vi "Config Parse.vi"(0 "Config File Path":path=path "C:/Automation/Configurations/VALEW.config", 11 "Error In":errorcluster) -> (4 "Pass/Fail?":bool, 6 "Report Text":string, 8 "VALEW_config":T1, 15 "Error Out":errorcluster)   [LabVIEW 2018, in "TL27.lvlib"]
uses:
  Projects/TL27.lvlib
  type defs/Config.ctl
  <vilib>/Utility/config.llb/Read Key (String).vi
  <vilib>/Utility/config.llb/Read Key (Boolean).vi
  <vilib>/Utility/config.llb/NI_LVConfig.lvlib
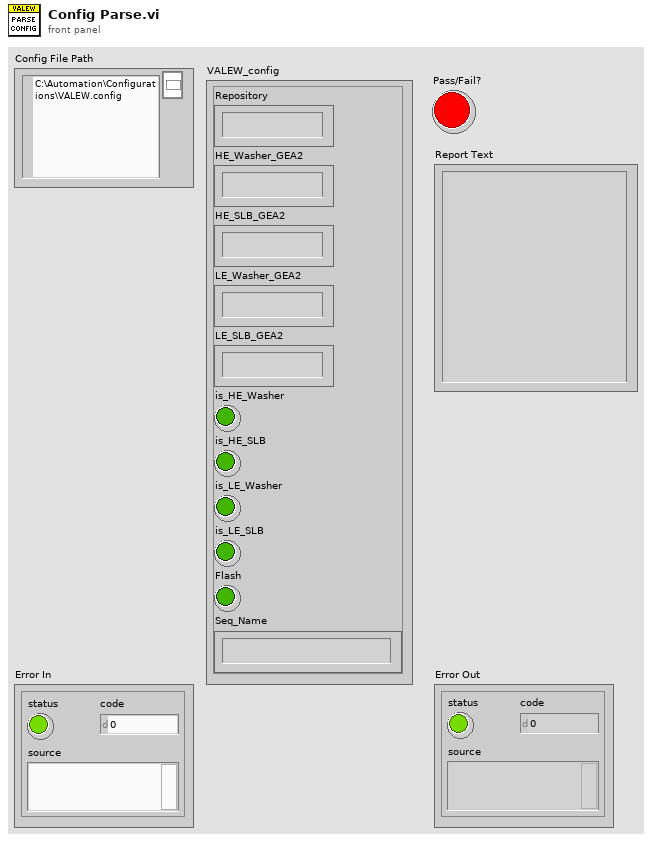
[diagram p1: front panel]
types:
  T1 = typedef "TL27.lvlib/Config.ctl" = cluster{"Repository":string, "HE_Washer_GEA2":string, "HE_SLB_GEA2":string, "LE_Washer_GEA2":string, "LE_SLB_GEA2":string, "is_HE_Washer":bool, "is_HE_SLB":bool, "is_LE_Washer":bool, "is_LE_SLB":bool, "Flash":bool, "Seq_Name":string}
  T2 = typedef "NI_LVConfig.lvlib/Config Data RefNum.ctl" = refnum<k1>
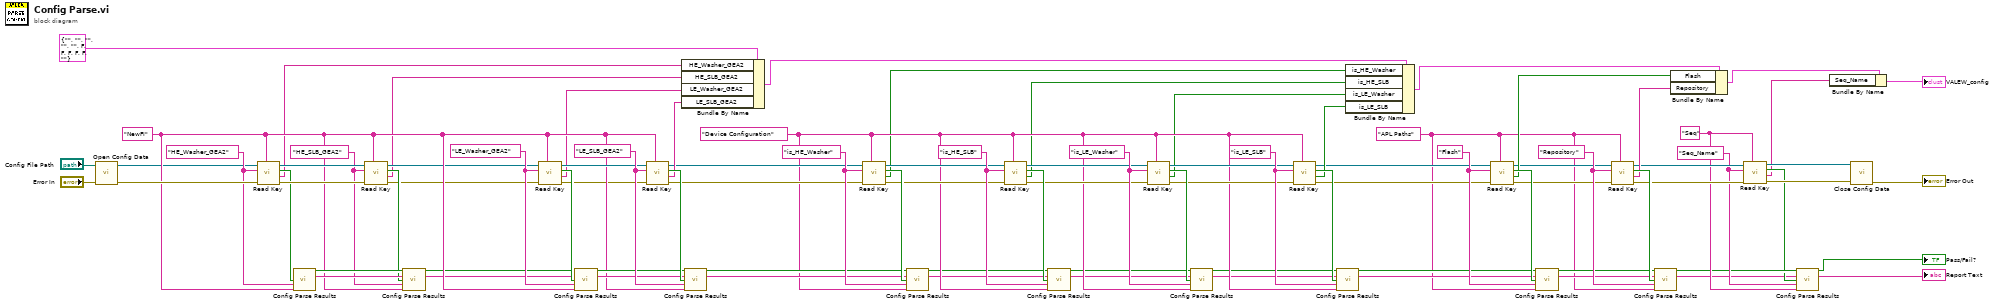
[diagram p0: block diagram]
diagram:
  w11 = "Seq_Name" ("key")
  w10 = "Seq" ("section")
  w23 = "Repository" ("key")
  w51 = "is_LE_SLB" ("key")
  w52 = "is_LE_Washer" ("key")
  w55 = "is_HE_SLB" ("key")
  w76 = "LE_SLB_GEA2" ("key")
  w71 = "LE_Washer_GEA2" ("key")
  w77 = "Flash" ("key")
  w7 = "APL Paths" ("section")
  w79 = "is_HE_Washer" ("key")
  w43 = "Device Configuration" ("section")
  w81 = "HE_SLB_GEA2" ("key")
  w86 = "HE_Washer_GEA2" ("key")
  w69 = "NewFI" ("section")
  n1 = call <vilib>:"Open Config Data.vi"("error in (no error)"="Error In", "configuration file path"="Config File Path") -> ("error out"=w89:errorcluster, "refnum"=w16:T2)  [unwired: 7 in, 1 out]
  n2 = call-poly <vilib>:"Read Key.vi"("section"=w69, "error in (no error)"=w89, "key"=w86, "refnum"=w16) -> ("error out"=w90:errorcluster, "value"=w63:string, "found?"=w85:bool, "refnum out"=w91:T2)  [unwired: 4 in]
  n3 = call "Config Parse Results.vi"("found?"=w85, "key"=w86, "section"=w69) -> ("Pass/Fail"=w84:bool, "Report Text"=w83:string)  [unwired: 11 in]
  n4 = call-poly <vilib>:"Read Key.vi"("section"=w69, "error in (no error)"=w90, "key"=w81, "refnum"=w91) -> ("error out"=w67:errorcluster, "value"=w62:string, "found?"=w82:bool, "refnum out"=w68:T2)  [unwired: 4 in]
  n5 = call "Config Parse Results.vi"("Previous Pass/Fail"=w84, "Previous Report Text"=w83, "found?"=w82, "key"=w81, "section"=w69) -> ("Pass/Fail"=w65:bool, "Report Text"=w64:string)  [unwired: 9 in]
  n6 = call-poly <vilib>:"Read Key.vi"("section"=w69, "error in (no error)"=w67, "key"=w71, "refnum"=w68) -> ("error out"=w66:errorcluster, "value"=w61:string, "found?"=w72:bool, "refnum out"=w70:T2)  [unwired: 4 in]
  n7 = call "Config Parse Results.vi"("Previous Pass/Fail"=w65, "Previous Report Text"=w64, "found?"=w72, "key"=w71, "section"=w69) -> ("Pass/Fail"=w73:bool, "Report Text"=w74:string)  [unwired: 9 in]
  n8 = call-poly <vilib>:"Read Key.vi"("section"=w69, "error in (no error)"=w66, "key"=w76, "refnum"=w70) -> ("error out"=w58:errorcluster, "value"=w60:string, "found?"=w75:bool, "refnum out"=w59:T2)  [unwired: 4 in]
  n9 = Bundle By Name(cluster=T1 {"Repository"="", "HE_Washer_GEA2"="", "HE_SLB_GEA2"="", "LE_Washer_GEA2"="", "LE_SLB_GEA2"="", "is_HE_Washer"=FALSE, "is_HE_SLB"=FALSE, "is_LE_Washer"=FALSE, "is_LE_SLB"=FALSE, "Flash"=FALSE, "Seq_Name"=""} ("VALEW_config"), "HE_Washer_GEA2"=w63, "HE_SLB_GEA2"=w62, "LE_Washer_GEA2"=w61, "LE_SLB_GEA2"=w60) -> (w33:T1)
  n10 = call "Config Parse Results.vi"("Previous Pass/Fail"=w73, "Previous Report Text"=w74, "found?"=w75, "key"=w76, "section"=w69) -> ("Pass/Fail"=w57:bool, "Report Text"=w56:string)  [unwired: 9 in]
  n11 = call-poly <vilib>:"Read Key.vi"("section"=w43, "error in (no error)"=w58, "key"=w79, "refnum"=w59) -> ("error out"=w47:errorcluster, "value"=w29:bool, "found?"=w80:bool, "refnum out"=w49:T2)  [unwired: 4 in]
  n12 = call "Config Parse Results.vi"("Previous Pass/Fail"=w57, "Previous Report Text"=w56, "found?"=w80, "key"=w79, "section"=w43) -> ("Pass/Fail"=w42:bool, "Report Text"=w41:string)  [unwired: 9 in]
  n13 = call-poly <vilib>:"Read Key.vi"("section"=w43, "error in (no error)"=w47, "key"=w55, "refnum"=w49) -> ("error out"=w46:errorcluster, "value"=w30:bool, "found?"=w54:bool, "refnum out"=w48:T2)  [unwired: 4 in]
  n14 = call "Config Parse Results.vi"("Previous Pass/Fail"=w42, "Previous Report Text"=w41, "found?"=w54, "key"=w55, "section"=w43) -> ("Pass/Fail"=w40:bool, "Report Text"=w39:string)  [unwired: 9 in]
  n15 = call-poly <vilib>:"Read Key.vi"("section"=w43, "error in (no error)"=w46, "key"=w52, "refnum"=w48) -> ("error out"=w45:errorcluster, "value"=w31:bool, "found?"=w53:bool, "refnum out"=w44:T2)  [unwired: 4 in]
  n16 = call "Config Parse Results.vi"("Previous Pass/Fail"=w40, "Previous Report Text"=w39, "found?"=w53, "key"=w52, "section"=w43) -> ("Pass/Fail"=w38:bool, "Report Text"=w37:string)  [unwired: 9 in]
  n17 = call-poly <vilib>:"Read Key.vi"("section"=w43, "error in (no error)"=w45, "key"=w51, "refnum"=w44) -> ("error out"=w28:errorcluster, "value"=w32:bool, "found?"=w50:bool, "refnum out"=w27:T2)  [unwired: 4 in]
  n18 = call "Config Parse Results.vi"("Previous Pass/Fail"=w38, "Previous Report Text"=w37, "found?"=w50, "key"=w51, "section"=w43) -> ("Pass/Fail"=w36:bool, "Report Text"=w35:string)  [unwired: 9 in]
  n19 = Bundle By Name(cluster=w33, "is_HE_Washer"=w29, "is_HE_SLB"=w30, "is_LE_Washer"=w31, "is_LE_SLB"=w32) -> (w26:T1)
  n20 = call-poly <vilib>:"Read Key.vi"("section"=w7, "error in (no error)"=w28, "key"=w77, "refnum"=w27) -> ("error out"=w18:errorcluster, "value"=w25:bool, "found?"=w78:bool, "refnum out"=w19:T2)  [unwired: 4 in]
  n21 = call "Config Parse Results.vi"("Previous Pass/Fail"=w36, "Previous Report Text"=w35, "found?"=w78, "key"=w77, "section"=w7) -> ("Pass/Fail"=w21:bool, "Report Text"=w20:string)  [unwired: 9 in]
  n22 = call-poly <vilib>:"Read Key.vi"("section"=w7, "error in (no error)"=w18, "key"=w23, "refnum"=w19) -> ("error out"=w15:errorcluster, "value"=w17:string, "found?"=w24:bool, "refnum out"=w13:T2)  [unwired: 4 in]
  n23 = call "Config Parse Results.vi"("Previous Pass/Fail"=w21, "Previous Report Text"=w20, "found?"=w24, "key"=w23, "section"=w7) -> ("Pass/Fail"=w9:bool, "Report Text"=w1:string)  [unwired: 9 in]
  n24 = Bundle By Name(cluster=w26, "Flash"=w25, "Repository"=w17) -> (w6:T1)
  n25 = call-poly <vilib>:"Read Key.vi"("section"=w10, "error in (no error)"=w15, "key"=w11, "refnum"=w13) -> ("error out"=w14:errorcluster, "value"=w5:string, "found?"=w8:bool, "refnum out"=w12:T2)  [unwired: 4 in]
  n26 = call "Config Parse Results.vi"("Previous Pass/Fail"=w9, "Previous Report Text"=w1, "found?"=w8, "key"=w11, "section"=w10) -> ("Pass/Fail"=→"Pass/Fail?":bool, "Report Text"=→"Report Text":string)  [unwired: 9 in]
  n27 = Bundle By Name(cluster=w6, "Seq_Name"=w5) -> (→"VALEW_config":T1)
  n28 = call <vilib>:"Close Config Data.vi"("error in (no error)"=w14, "refnum"=w12) -> ("error out"=→"Error Out":errorcluster)  [unwired: 8 in, 1 out]
